vi "Display.vi"(8 "error in":errorcluster, 11 "Gif - One Button in":refnum<class "SVG - One Button.lvclass">) -> (0 "error out":errorcluster, 3 "Gif - One Button out":refnum<class "SVG - One Button.lvclass">)   [LabVIEW 2019, in "Pop-Up.lvlib" / "SVG - One Button.lvclass"]
doc: "This is the override method required for each child of the pop up class. It is the pop up that will display to the user.\n\nTo extend this function, create a child class of the pop up class. Then create an override method for this VI. <b>Display.vi</b> is a protected function, therefore it cannot be called in a main application. This VI must be called by a caller function. See one of the standard pop-ups for a setup example.\n\n<b>Code Developed By:</b>\nDaniel Coons\nTechnology Service Corporation\n1983 S Liberty Drive\nBloomington, IN 47403\nPhone: 812 558-7100\ndaniel.coons@tsc.com\nwww.tsc.com/atcs"
uses:
  SVG - One Button.lvclass
  C:/Development/tsc-pop-up/Popup/Popup.lvclass
  Popup/Popup.lvclass/Popup.ctl
  Popup/Data Member Access/Read Theme.vi
  Theme/Theme.lvclass
  Popup/Popup.lvclass
  user32.dll
panel:
  out "header":bool
  out "Message":string
  out "2D Picture":picture
  in  "OK":bool
  # "This VI displays the popup"
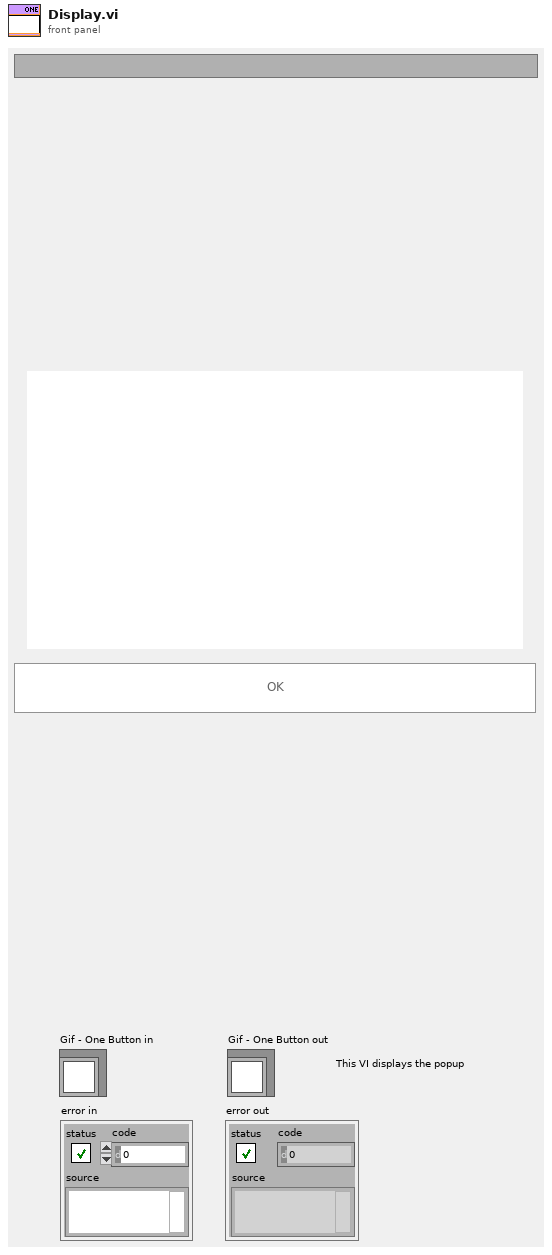
[diagram p1: front panel]
types:
  T1 = typedef "LVPoint32TypeDef.ctl" = cluster{"Horizontal":i32, "Vertical":i32}
  T2 = typedef "LVPositionTypeDef.ctl" = cluster{"Left":i32, "Top":i32}
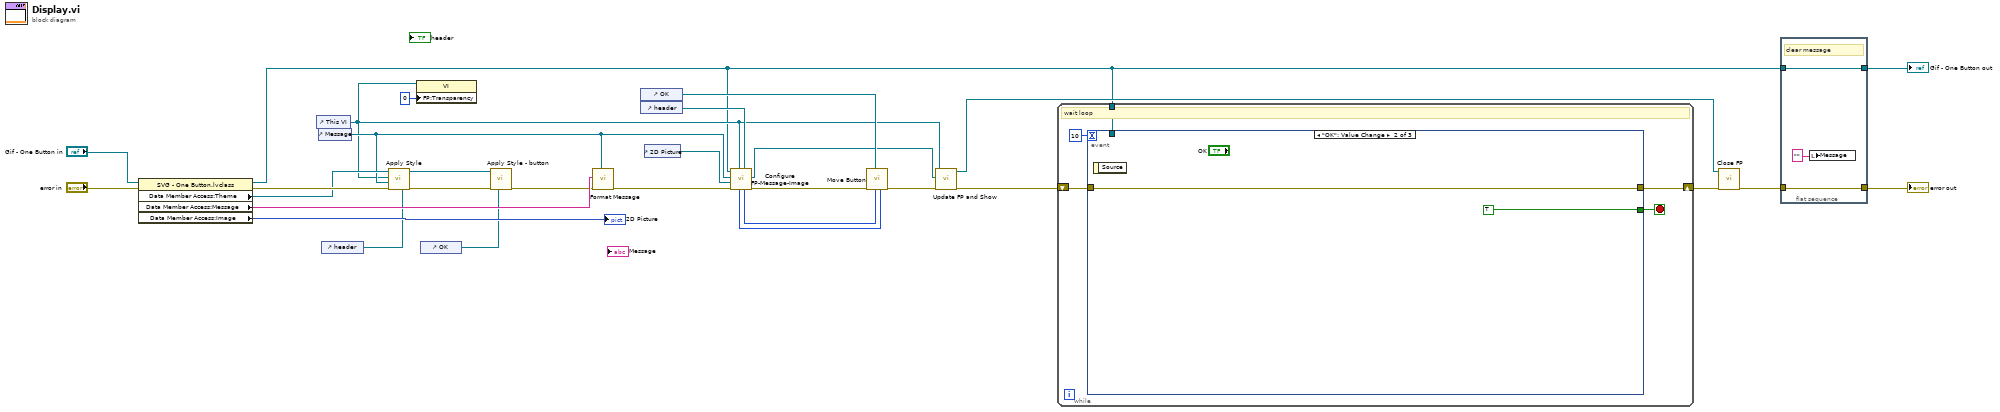
[diagram p0: block diagram]
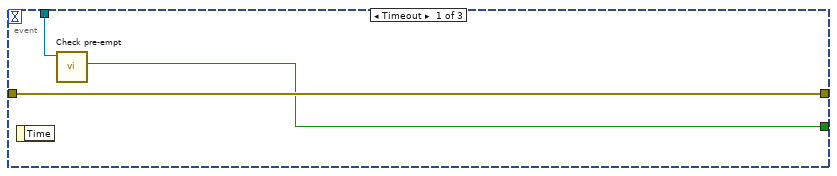
[diagram p2: hidden frame]
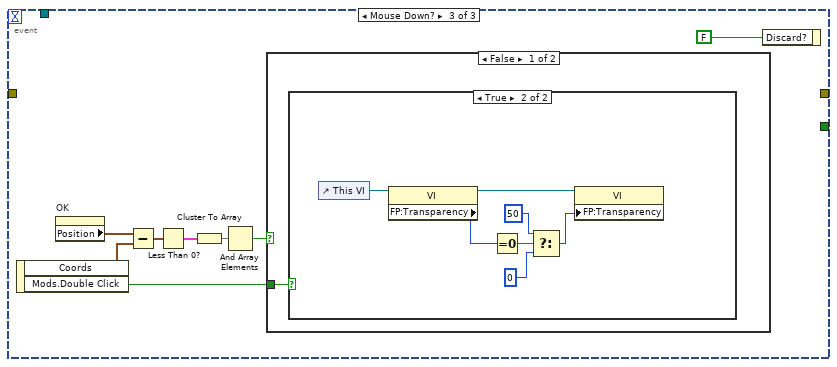
[diagram p3: hidden frame]
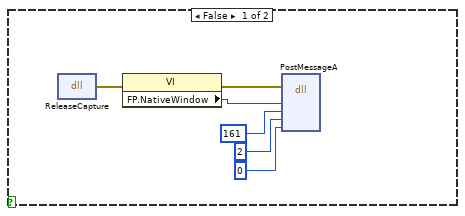
[diagram p4: hidden frame]
diagram:
  n1 = property class="SVG - One Button.lvclass"(reference="Gif - One Button in", error in="error in") -> (reference out=w1:refnum<class "SVG - One Button.lvclass">, error out=w30:errorcluster, "Data Member Access:Theme"=w25:refnum<class "Theme.lvclass">, "Data Member Access:Message"=w23:string, "Data Member Access:Image"=→"2D Picture":picture)
  n2 = control-ref of="This VI"() -> (w7:refnum<vi>)
  n3 = control-ref of="Message"() -> (w19:refnum<vi>)
  n4 = control-ref of="header"() -> (w11:refnum<vi>)
  n5 = call "Apply Style.vi"("header ref"=w11, "error in (no error)"=w30, "message ref"=w19, "pop up ref"=w7, "Theme in"=w25) -> ("error out"=w13:errorcluster, "Theme out"=w22:refnum<class "Theme.lvclass">)  [unwired: 5 in]
  n6 = property class="VI"(reference=w7, "FP:Transparency"=u8 0 ("Front Panel Window:Transparency")) -> ()  [unwired: 1 in, 2 out]
  n7 = control-ref of="OK"() -> (w21:refnum<vi>)
  n8 = call "Apply Style - button.vi"("button ref"=w21, "error in (no error)"=w13, "Theme in"=w22) -> ("error out"=w12:errorcluster)  [unwired: 7 in, 1 out]
  n9 = call "Format Message.vi"("formatted string"=w19, "error in"=w12, "String Input"=w23) -> ("error out"=w9:errorcluster)  [unwired: 7 in, 1 out]
  n10 = control-ref of="OK"() -> (w20:refnum<vi>)
  n11 = control-ref of="header"() -> (w14:refnum<vi>)
  n12 = control-ref of="2D Picture"() -> (w18:refnum<vi>)
  n13 = call "Configure FP-Message-Image.vi"("header ref"=w14, "Pop Up ref"=w7, "error in (no error)"=w9, "Image ref"=w18, "Message ref"=w19, "Popup in"=w1) -> ("error out"=w10:errorcluster, "Panel Ref"=w15:refnum<vi>, "Panel Width"=w17:i32, "Panel Height"=w16:i32)  [unwired: 1 in, 1 out]
  n14 = call "Move Button.vi"("Panel Height"=w16, "Panel Width"=w17, "Button"=w20, "Error In"=w10) -> ("Error Out"=w29:errorcluster)  [unwired: 6 in, 1 out]
  n15 = call "Update FP and Show.vi"("error in (no error)"=w29, "Panel Ref"=w15, "VI in"=w7) -> ("error out"=w26:errorcluster, "VI out"=w8:refnum<vi>)  [unwired: 7 in]
  n16 = while {
    shift-right: [w35] -> w28
    shift-left: w26 -> [w34]
    tunnel: w1 -> [w32]
    stop <- w31 stop-if-true
    # "wait loop"
    n17 = event shown="[1] \"OK\": Value Change" {
      selector: _ -> [_ _ _]
      dyn-events: _ -> [_ _ _]
      timeout: 10 -> [_ _ _]
      tunnel: w34 -> [w38 w40 _]
      tunnel: [w38 w40 _] -> w35
      tunnel: [w36 TRUE _] -> w31
      tunnel: w32 -> [w37 _ _]
      event Timeout {
        n18 = event-data() -> ()  [unwired: 1 in, 1 out]
        n19 = call "Check pre-empt.vi"("_Popup in"=w37) -> ("Pre-empted?"=w36:bool)  [unwired: 8 in, 2 out]
      }
      event "OK": Value Change {
        n20 = event-data() -> ()  [unwired: 1 in, 1 out]
      }
      event Mouse Down? {
        n21 = event-data() -> ("Coords"=w41:T1, "Mods.Double Click"=w42:bool)  [unwired: 1 in]
        n22 = property on="OK" class="Bool"() -> ("Position"=w43:T2)  [unwired: 2 in, 2 out]
        n23 = Subtract(x=w43, y=w41) -> (x-y=w44:T2)
        n24 = Less Than 0?(x=w44) -> (x < 0?=w45:cluster{"Left":bool, "Top":bool})
        n25 = Cluster To Array(cluster=w45) -> (array=w46:bool[])
        n26 = And Array Elements(Boolean array=w46) -> (logical AND=w47:bool)
        n27 = case shown="False" w47 {
          tunnel: w42 -> [w49 _]
          frame False {
            n28 = case shown="True" w49 {
              frame False {
                n29 = dll-call lib="user32.dll" fn="ReleaseCapture"() -> (error out=w53:errorcluster)  [unwired: 4 in, 1 out]
                n30 = property class="VI"(error in=w53) -> (error out=w54:errorcluster, "FP.NativeWindow"=w55:u64)  [unwired: 1 in, 1 out]
                n31 = dll-call lib="user32.dll" fn="PostMessageA"(error in=w54, "hWnd"=w55, "Msg"=161, "wParam"=2, "lParam"=0) -> ()  [unwired: 7 in, 2 out]
              }
              frame True {
                n32 = control-ref of="This VI"() -> (w62:refnum<vi>)
                n33 = property class="VI"(reference=w62) -> (reference out=w60:refnum<vi>, "FP:Transparency"=w61:u8)  [unwired: 1 in, 1 out]
                n34 = Equal To 0?(x=w61) -> (x = 0?=w59:bool)
                n35 = Select(t=u8 50, s=w59, f=u8 0) -> (s? t:f=w58:u8)
                n36 = property class="VI"(reference=w60, "FP:Transparency"=w58) -> ()  [unwired: 1 in, 2 out]
              }
            }
          }
          frame True {
          }
        }
        n37 = event-data("Discard?"=FALSE) -> ()  [unwired: 1 in, 1 out]
      }
    }
  }
  n38 = call "Close FP.vi"("error in (no error)"=w28, "VI in"=w8) -> ("error out"=w27:errorcluster)  [unwired: 9 in]
  n39 = flat-sequence {
    tunnel: w27 -> [w65]
    tunnel: [w65] -> w2
    tunnel: w1 -> [w64]
    tunnel: [w64] -> w3
    frame #0 {
      # "clear message"
      n40 = local write "Message"("" ("Message")) -> ()
    }
  }
  "error out" <- w2
  "Gif - One Button out" <- w3
